vi "Common_Socket_FWUgrade_Cmd_Sub_VI.vi"(0 "TCP_IN":refnum<k5>, 1 "Response ID 1":u8, 7 "FW Message ID":i32, 9 "FW Message Length":i32, 11 "error in":errorcluster) -> (4 "connection ID":refnum<k5>, 6 "Data Response":string, 10 "error out":errorcluster, 15 "Pass":string)   [LabVIEW 2017]
panel:
  out "*(type *) &x":u8
  out "bytes written":i32
  # "Refrence:"
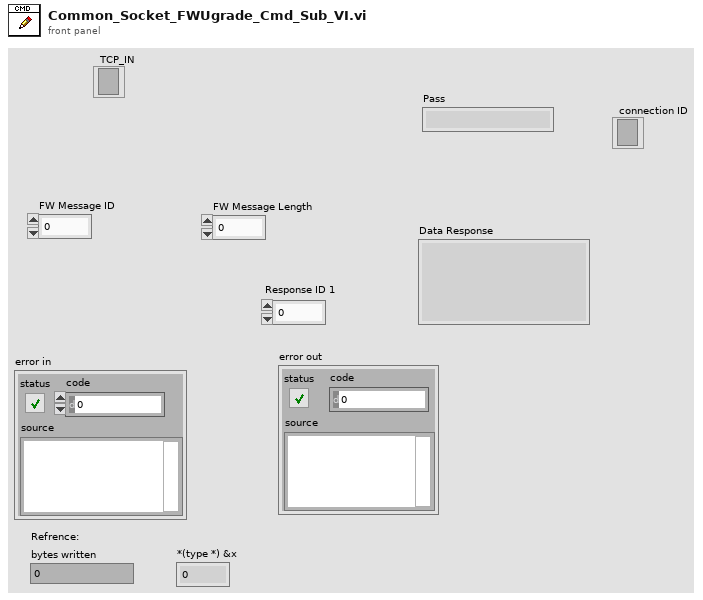
[diagram p1: front panel]
types:
  T1 = enum16{"big-endian, network order", "native, host order", "little-endian"}
  T2 = cluster{"FW Message Length":i32, "FW Message ID":i32}
  T3 = enum16{"Standard", "Buffered", "CRLF", "Immediate"}
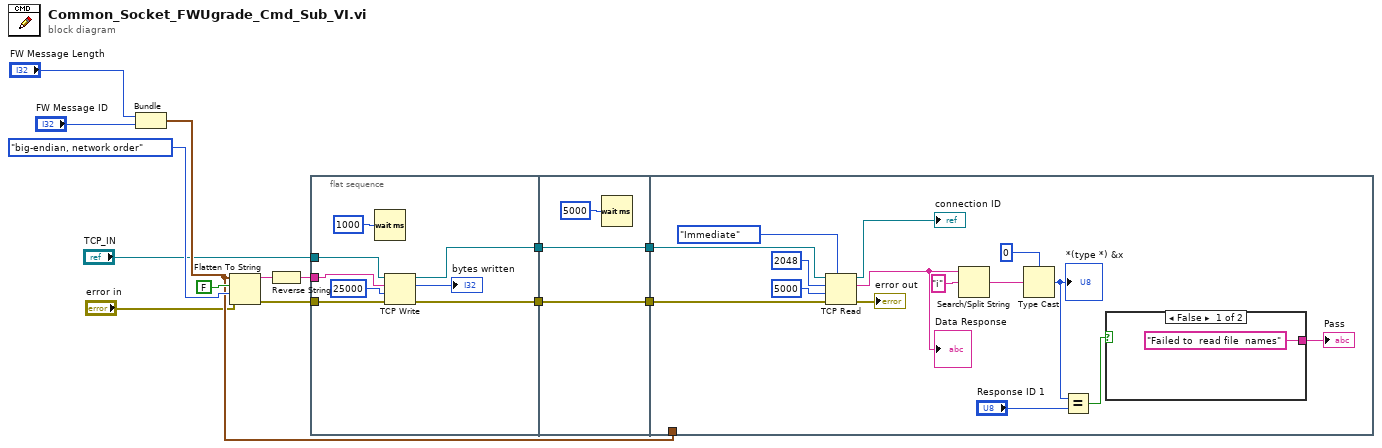
[diagram p0: block diagram]
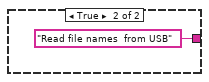
[diagram p2: hidden frame]
diagram:
  n1 = Bundle("FW Message Length"="FW Message Length", "FW Message ID"="FW Message ID") -> (w3:T2)  [unwired: 1 in]
  n2 = Flatten To String(anything=w3, prepend array or string size? (T)=FALSE, byte order (0:big-endian, network order)=T1."big-endian, network order", error in (no error)="error in") -> (data string=w6:string, error out=w7:errorcluster)  [unwired: 1 out]
  n3 = Reverse String(1:w6) -> (0:w5:string)
  n4 = flat-sequence {
    tunnel: [w20] -> w14
    tunnel: [w19] -> w13
    tunnel: w7 -> [w18]
    tunnel: w5 -> [w17]
    tunnel: "TCP_IN" -> [w15]
    tunnel: [w24] -> w12
    tunnel: w14 -> [w24]
    tunnel: [w23] -> w11
    tunnel: w13 -> [w23]
    tunnel: w12 -> [w40]
    tunnel: w11 -> [w39]
    tunnel: w3 -> [_]
    frame #0 {
      n5 = Wait (ms)(milliseconds to wait=u32 1000) -> ()  [unwired: 1 out]
      n6 = TCP Write(connection ID=w15, data in=w17, error in (no error)=w18, 9:25000 ("timeout ms (25000)")) -> (connection ID out=w20:refnum<k5>, bytes written=→"bytes written":i32, error out=w19:errorcluster)
    }
    frame #1 {
      n7 = Wait (ms)(milliseconds to wait=u32 5000) -> ()  [unwired: 1 out]
    }
    frame #2 {
      n8 = TCP Read(connection ID=w40, bytes to read=2048, error in (no error)=w39, 7:T3."Immediate" ("mode (standard)"), 9:5000 ("timeout ms (25000)")) -> (connection ID out=→"connection ID":refnum<k5>, data out=w28:string, error out=→"error out":errorcluster)
      "Data Response" <- w28
      n9 = Search/Split String(string=w28, search string/char (-)="i") -> (match + rest of string=w30:string)  [unwired: 1 in, 2 out]
      n10 = Type Cast(type=u8 0, x=w30) -> (*(type *) &x=w34:u8)
      "*(type *) &x" <- w34
      n11 = Equal?(x=w34, y="Response ID 1") -> (x = y?=w29:bool)
      n12 = case shown="False" w29 {
        tunnel: ["Failed to  read file  names" "Read file names  from USB"] -> w27
        frame False {
        }
        frame True {
        }
      }
      "Pass" <- w27
    }
  }
